vi "Request Task Add.vi"(8 "error in (no error)":errorcluster, 9 "Task":refnum<class "Task.lvclass">, 10 "index":i32, 11 "Comm Interface in":refnum<class "Comm Interface.lvclass">) -> (0 "error out":errorcluster, 3 "Comm Interface out":refnum<class "Comm Interface.lvclass">)   [LabVIEW 2017, in "Comm Interface.lvlib" / "Comm Interface.lvclass"]
uses:
  Comm Interface.lvclass
  Message Interface/Command/Command.lvclass
  Task Interface/Task/Task.lvclass
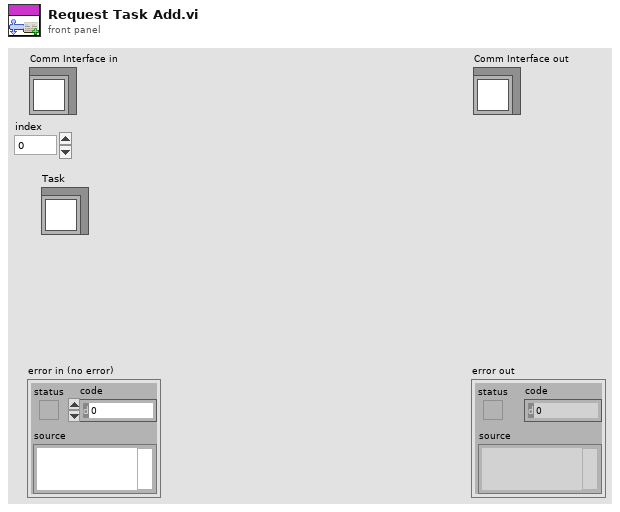
[diagram p1: front panel]
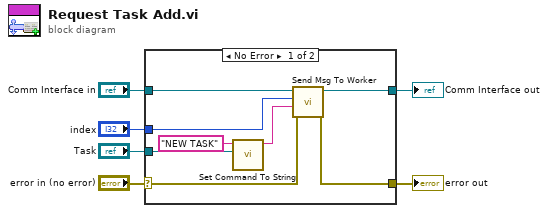
[diagram p0: block diagram]
diagram:
  n1 = case shown="No Error" "error in (no error)" {
    selector: "error in (no error)" -> [w8 w16]
    tunnel: [w7 w16] -> w5
    tunnel: [w12 w15] -> w3
    tunnel: "Comm Interface in" -> [w13 w15]
    tunnel: "Task" -> [w10 _]
    tunnel: "index" -> [w9 _]
    frame No Error {
      n2 = call "Set Command To String.vi"("Arguments"=w10, "Command"="NEW TASK") -> ("data string"=w11:string)  [unwired: 9 in]
      n3 = call "Send Msg To Worker.vi"("error in (no error)"=w8, "Message"=w11, "index"=w9, "Comm Interface in"=w13) -> ("error out"=w7:errorcluster, "Comm Interface out"=w12:refnum<class "Comm Interface.lvclass">)  [unwired: 6 in]
    }
    frame Error {
    }
  }
  "error out" <- w5
  "Comm Interface out" <- w3
